vi "example 3 - subpanel2.vi"() -> ()   [LabVIEW 2020]
panel:
  out "Plot":dbl[](graph)
  in  "Random":bool
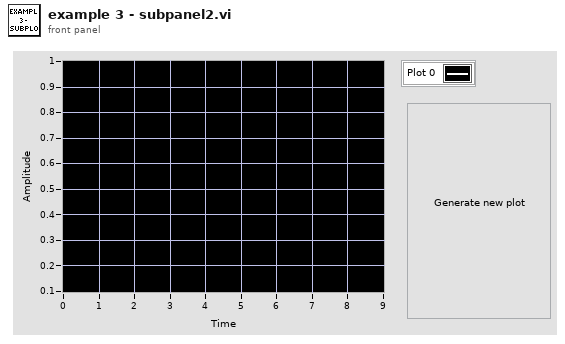
[diagram p1: front panel]
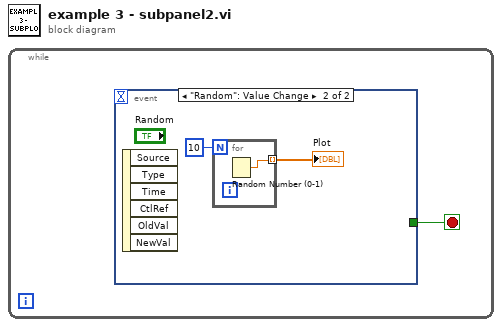
[diagram p0: block diagram]
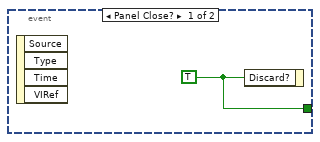
[diagram p2: hidden frame]
diagram:
  n1 = while {
    stop <- w1 stop-if-true
    n2 = event shown="[1] \"Random\": Value Change" {
      selector: _ -> [_ _]
      dyn-events: _ -> [_ _]
      timeout: _ -> [_ _]
      tunnel: [w2 _] -> w1
      event Panel Close? {
        w2 = TRUE
        n3 = event-data() -> ()  [unwired: 1 in, 4 out]
        n4 = event-data("Discard?"=w2) -> ()  [unwired: 1 in, 1 out]
      }
      event "Random": Value Change {
        n5 = event-data() -> ()  [unwired: 1 in, 6 out]
        n6 = for {
          N: 10 -> [_]
          tunnel: [w5] -> w3 mode=indexing
          n7 = Random Number (0-1)() -> (number: 0 to 1=w5:dbl)
        }
        "Plot" <- w3
      }
    }
  }
